vi "SlaveDoneUpdate.vi"(9 "shared index":i32, 11 "shared variable":refnum<k21>) -> ()   [LabVIEW 2018, in "TektronikNetwork.lvlib"]
uses:
  Tektronik3102/TektronikNetwork.lvlib
  Shared program Control/MasterStatus.ctl
  Shared program Control/MySharedVariables.lvlib
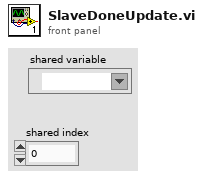
[diagram p1: front panel]
types:
  T1 = typedef "MySharedVariables.lvlib/MasterStatus.ctl" = cluster{"Camera done":bool, "Tektronik done":bool, "Motors done":bool, "Gage":bool}[]
  T2 = cluster{"Camera done":bool, "Tektronik done":bool, "Motors done":bool, "Gage":bool}
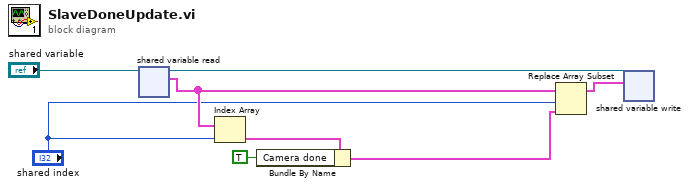
[diagram p0: block diagram]
diagram:
  n1 = shared-variable-read("shared variable") -> (w8:refnum<k21>, w6:T1)  [unwired: 1 in, 2 out]
  n2 = Index Array(array=w6, index="shared index") -> (element=w4:T2)
  n3 = Bundle By Name(cluster=w4, "Camera done"=TRUE) -> (w2:T2)
  n4 = Replace Array Subset(array=w6, new element=w2, index="shared index") -> (w7:T1)
  n5 = shared-variable-write(w8, w7) -> ()  [unwired: 1 in, 2 out]
